vi "Read_K7DRAMFIFO.vi"(6 "Ready for Output":bool, 11 "DRAM FIFO Ref In":refnum<class "K7 DRAM FIFO.lvclass">) -> (1 "Output Valid":bool, 2 "Element":bool[](array[boolean]), 3 "DRAM FIFO Ref Out":refnum<class "K7 DRAM FIFO.lvclass">)   [LabVIEW 2014, in "K7 DRAM FIFO.lvclass"]
doc: "Reads and removes the oldest element from the DRAM FIFO\n\n<B>Inputs</B>\n<B>DRAM FIFO Ref In</B> specifies the FIFO. \n<B>Ready for Output</B>specifies whether downstream nodes are ready for this node to return a new value. The default is TRUE. Use a Feedback Node to wire the Ready for Input output of a downstream node to this input of the current node. \n\n<B>Outputs</B>\n<B>DRAM FIFO Ref Out</B> specifies the FIFO.\n<B>Element</B> returns the oldest data element in the FIFO\n<B>Output Valid</B> returns TRUE if this node has computed a result that downstream nodes can use. Wire this output to the Input Valid input of a downstream node to transfer data from this node to the downstream node. \n\n<B>Detailed Help</B>\nThe DRAM FIFO Ref can come from Write DRAM FIFO if both are used in the same clock domain. Otherwise, the reference should originate from Create DRAM FIFO. \n\nIf Ready for Output is FALSE during a given cycle, the Output Valid terminal returns FALSE during the given cycle. \n\nThe Data Manipulation library has functions that assist with converting the boolean array back into the original data type."
uses:
  K7 DRAM FIFO.lvclass
  <vilib>/rvi/DataTransferAndStorage/Container/XNode/niFpgaContainer.xnode
  <vilib>/rvi/FIFO/Fifo_Resource/niFpgaFifoEmulationRefIn.vi
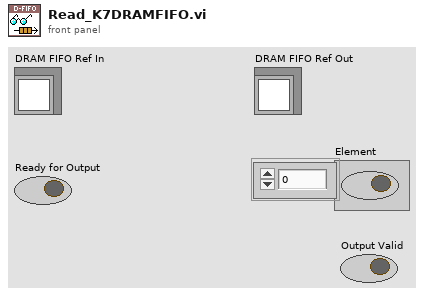
[diagram p1: front panel]
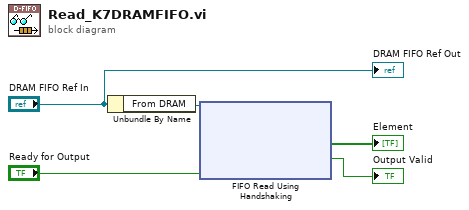
[diagram p0: block diagram]
diagram:
  n1 = Unbundle By Name("DRAM FIFO Ref In") -> ("From DRAM"=w5:refnum<k21>)
  n2 = xnode "FIFO Read Using Handshaking"("Ready for Output"="Ready for Output", "FIFO In"=w5) -> ("Element"=→"Element":bool[], "Output Valid"=→"Output Valid":bool)  [unwired: 1 out]
  "DRAM FIFO Ref Out" <- "DRAM FIFO Ref In"
